vi "Vision Logic.vi"(8 "X-2":i32, 11 "X-1":i32) -> ()   [LabVIEW 2016]
uses:
  <vilib>/Rock Robotics/WPI/Utilities/WPI_GetSetVariantRefNum.vi
  <vilib>/Rock Robotics/WPI/RobotDrive/WPI_RobotDriveArcadeDrive_RatioCurve.vi
panel:
  in  "Y-2":i32
  in  "Y-1":i32
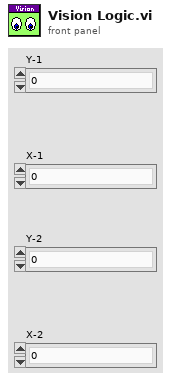
[diagram p1: front panel]
types:
  T1 = typedef "WPI_RobotDriveDevRef.ctl" = cluster{"DevStatus":errorcluster, "Motors[]":T2[], "Square Inputs":bool, "Max Output":dbl}
  T2 = typedef "WPI_MotorControlDeviceRef.ctl" = cluster{"DeviceStatus":errorcluster, "Type":T3, "PWM":cluster{"PWM Channel":T4, "DeadBand":T5}, "CAN":cluster{"Device Number":u8, "SetOutput VI Ref":variant, "GetOutput VI Ref":variant, "Enable VI Ref":variant, "Disable VI Ref":variant, "Data":variant}, "Invert":bool}
  T3 = typedef "WPI_MotorControlType.ctl" = enum16{"PWM", "CAN"}
  T4 = typedef "FPGA_DIOPWMChannel.ctl" = enum8{"PWM 0", "PWM 1", "PWM 2", "PWM 3", "PWM 4", "PWM 5", "PWM 6", "PWM 7", "PWM 8", "PWM 9", "PWM MXP 0", "PWM MXP 1", "PWM MXP 2", "PWM MXP 3", "PWM MXP 4", "PWM MXP 5", "PWM MXP 6", "PWM MXP 7", "PWM MXP 8", "PWM MXP 9", "Invalid"}
  T5 = typedef "WPI_PWMDeadband.ctl" = cluster{"Name":string, "maxPositivePwm":i32, "minPositivePwm":i32, "centerPwm":i32, "maxNegativePwm":i32, "minNegativePwm":i32, "angularRange":u16}
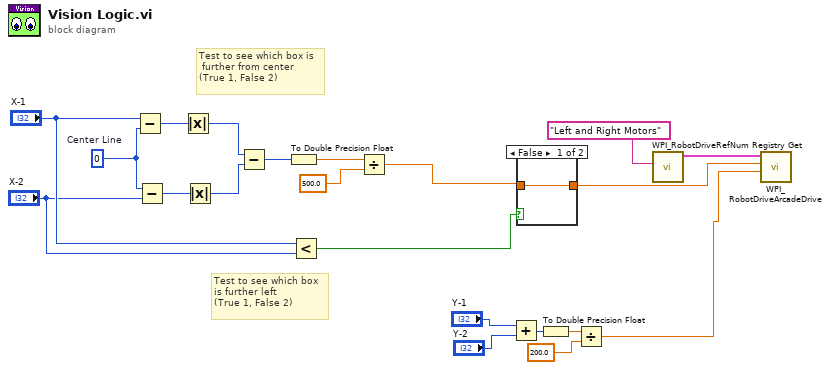
[diagram p0: block diagram]
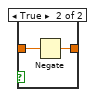
[diagram p2: hidden frame]
diagram:
  w19 = 0  # Center Line
  # "Test to see which box\nis further left\n(True 1, False 2)"
  # "Test to see which box is\n further from center \n(True 1, False 2)"
  n1 = Subtract(x="X-1", y=w19) -> (x-y=w21:i32)
  n2 = Subtract(x=w19, y="X-2") -> (x-y=w20:i32)
  n3 = Absolute Value(x=w21) -> (abs(x)=w18:i32)
  n4 = Absolute Value(x=w20) -> (abs(x)=w17:i32)
  n5 = Subtract(x=w18, y=w17) -> (x-y=w12:i32)
  n6 = To Double Precision Float(number=w12) -> (double precision float=w14:dbl)
  n7 = Less?(x="X-1", y="X-2") -> (x < y?=w8:bool)
  n8 = Divide(x=w14, y=500.0) -> (x/y=w9:dbl)
  n9 = Add(x="Y-1", y="Y-2") -> (x+y=w4:i32)
  n10 = case shown="False" w8 {
    tunnel: w9 -> [w22 w24]
    tunnel: [w22 w23] -> w7
    frame False {
    }
    frame True {
      n11 = Negate(x=w24) -> (-x=w23:dbl)
    }
  }
  n12 = To Double Precision Float(number=w4) -> (double precision float=w3:dbl)
  n13 = Divide(x=w3, y=200.0) -> (x/y=w1:dbl)
  n14 = call <vilib>:"WPI_RobotDriveRefNum Registry Get.vi"("refnum name"="Left and Right Motors") -> ("RobotDriveDevRef"=w10:T1)  [unwired: 9 in, 1 out]
  n15 = call-poly <vilib>:"WPI_RobotDriveArcadeDrive.vi"("Y axis value (Speed)"=w1, "X axis value (Curve)"=w7, "RobotDriveDevRef"=w10) -> ()  [unwired: 6 in, 3 out]
